vi "Check_Initial_States.vi"(9 "CmbBox Refnum":refnum<vi>, 10 "Str Refnum":refnum<vi>, 11 "Boolean in":refnum<vi>) -> ()   [LabVIEW 2017]
uses:
  97e3525f-9c52-4a5f-8e12-8558b348f06f.vi
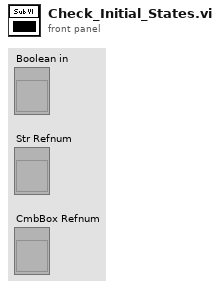
[diagram p1: front panel]
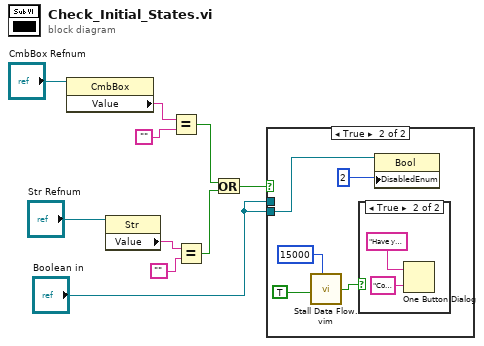
[diagram p0: block diagram]
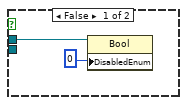
[diagram p2: hidden frame]
diagram:
  n1 = property on="Property Node" class="CmbBox"(reference="CmbBox Refnum") -> ("Value"=w6:string)  [unwired: 1 in, 2 out]
  n2 = property on="Property Node" class="Str"(reference="Str Refnum") -> ("Value"=w4:string)  [unwired: 1 in, 2 out]
  n3 = Equal?(x=w6, y="") -> (x = y?=w9:bool)
  n4 = Equal?(x=w4, y="") -> (x = y?=w8:bool)
  n5 = Or(x=w9, y=w8) -> (x .or. y?=w10:bool)
  n6 = case shown="True" w10 {
    tunnel: "Boolean in" -> [w11 _]
    tunnel: "Boolean in" -> [_ w13]
    frame False {
      n7 = property on="Property Node" class="Bool"(reference=w11, "DisabledEnum"=0) -> ()  [unwired: 1 in, 2 out]
    }
    frame True {
      n8 = call "Stall Data Flow.vim"("value in"=TRUE, "milliseconds to wait"=15000) -> ("value out"=w16:bool)  [unwired: 1 out]
      n9 = case shown="True" w16 {
        frame False {
        }
        frame True {
          n10 = One Button Dialog(message="Have you entered the Name/ID of the Subject?\n\nHave you entered the Location to save the data?\n\nHave you entered where you are measuring Skin Tenting?\n\nIn order to start acquisition, please fill all these fields.", button name ("OK")="Continue") -> ()  [unwired: 1 out]
        }
      }
      n11 = property on="Property Node" class="Bool"(reference=w13, "DisabledEnum"=2) -> ()  [unwired: 1 in, 2 out]
    }
  }
